vi "LocalOrGlobalTarget.vi"(6 "Direction":enum16{" +", " - "}(ring)=enum." - ", 11 "Target":T1) -> (3 "Adjusted Target":T1)   [LabVIEW 2009]
uses:
  Target.ctl
  Data Access Objects/Metadata/LBCB Number.ctl
  Global Data/Cartesian Measurment Actions.ctl
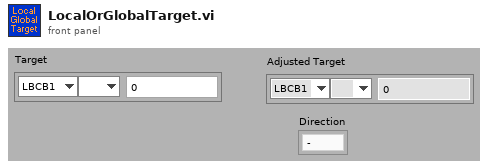
[diagram p1: front panel]
types:
  T1 = typedef "Target.ctl" = cluster{"LBCB Number":T2, "DOF Vectors":enum16{" ", "Dx", "Dy", "Dz", "Rx", "Ry", "Rz", "Fx", "Fy", "Fz", "Mx", "My", "Mz"}, "Amount":dbl}
  T2 = typedef "LBCB Number.ctl" = enum16{"LBCB1", "LBCB2"}
  T3 = typedef "Cartesian Measurment Actions.ctl" = enum16{"Set Data", "Get", "Init", "Set Offsets"}
  T4 = enum16{" ", "Dx", "Dy", "Dz", "Rx", "Ry", "Rz", "Fx", "Fy", "Fz", "Mx", "My", "Mz"}
  T5 = typedef "Cartesian Data Type.ctl" = cluster{"Displacements":dbl[], "Forces":dbl[], "Displacement Commands":dbl[]}
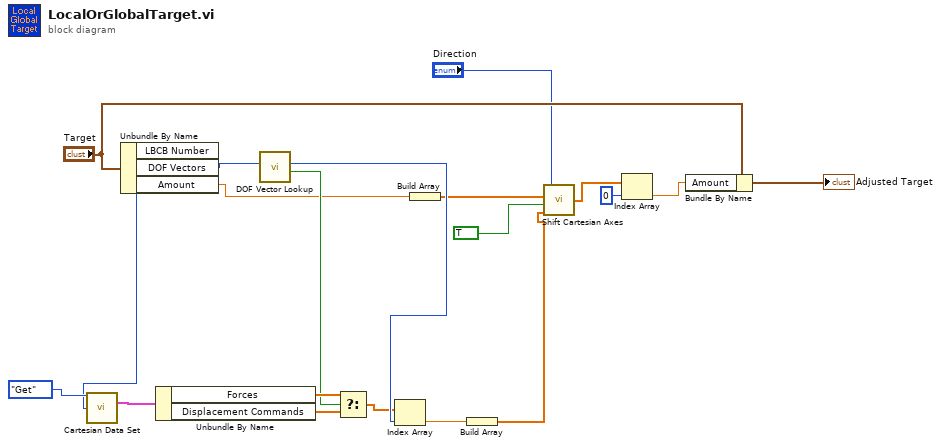
[diagram p0: block diagram]
diagram:
  n1 = Unbundle By Name("Target") -> ("LBCB Number"=w11:T2, "DOF Vectors"=w20:T4, "Amount"=w8:dbl)
  n2 = call "Cartesian Data Set.vi"("Measurement Actions"=Cartesian_Measurment_Actions."Get", "LBCB Selected"=w11) -> ("Cartesian Data Offsets Out"=w10:T5)  [unwired: 4 in, 9 out]
  n3 = Unbundle By Name(w10) -> ("Forces"=w14:dbl[], "Displacement Commands"=w13:dbl[])
  n4 = call "DOF Vector Lookup.vi"("DOF Vectors"=w20) -> ("IsForce"=w12:bool, "Index"=w17:u32)  [unwired: 9 out]
  n5 = Select(t=w14, s=w12, f=w13) -> (s? t:f=w9:dbl[])
  n6 = Index Array(array=w9, index=w17) -> (element=w6:dbl)
  n7 = Build Array(w8) -> (w7:dbl[])
  n8 = Build Array(w6) -> (w5:dbl[])
  n9 = call "Shift Cartesian Axes.vi"("Coordianate Offset"=w5, "Coordinate Switch"=TRUE, "Coordianate Input"=w7, "Direction"="Direction") -> ("Coordianate Output"=w4:dbl[])
  n10 = Index Array(array=w4, index=0) -> (element=w3:dbl)
  n11 = Bundle By Name(cluster="Target", "Amount"=w3) -> (→"Adjusted Target":T1)
